vi "Destroy User Events.vi"(11 "UI Template in":refnum<class "ACQ Generador.lvclass">) -> (3 "UI Template out":refnum<class "ACQ Generador.lvclass">)   [LabVIEW 2020, in "ACQ Generador.lvlib" / "ACQ Generador.lvclass"]
uses:
  ACQ Generador.lvclass
  ACQ Generador.lvclass/ACQ Generador.ctl
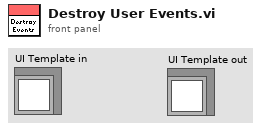
[diagram p1: front panel]
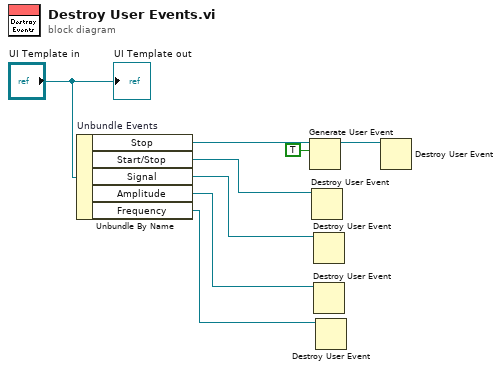
[diagram p0: block diagram]
diagram:
  n1 = Unbundle By Name "Unbundle Events"("UI Template in") -> ("Stop"=w6:refnum<user-event>, "Start/Stop"=w4:refnum<user-event>, "Signal"=w3:refnum<user-event>, "Amplitude"=w2:refnum<user-event>, "Frequency"=w1:refnum<user-event>)
  n2 = Generate User Event(user event=w6, event data cluster=TRUE ("event data")) -> (user event out=w7:refnum<user-event>)  [unwired: 2 in, 1 out]
  n3 = Destroy User Event(user event=w4) -> ()  [unwired: 1 in, 1 out]
  n4 = Destroy User Event(user event=w3) -> ()  [unwired: 1 in, 1 out]
  n5 = Destroy User Event(user event=w2) -> ()  [unwired: 1 in, 1 out]
  n6 = Destroy User Event(user event=w1) -> ()  [unwired: 1 in, 1 out]
  n7 = Destroy User Event(user event=w7) -> ()  [unwired: 1 in, 1 out]
  "UI Template out" <- "UI Template in"
